vi "Emballage_BDD_GVF_DATACMD.vi"(0 "SetGet":T2=enum."get", 1 "Quantité de la commande IN":string, 5 "Cmde_Interne? IN":bool, 7 "Annuler new série (T=OK) IN":bool, 9 "No commande FAS IN":string, 11 "Error in":errorcluster caption="Error in (no error)", 12 "DATA cmde IN":T1={"n°article FAS"="12-216E-01-25 F120023 500mA 10ohm", "n° cmde FAS"="R03844/08-01.01.01", "quantité cmde"="4", "ID LIG cmde"="225540", "n° cmde client"="120565              ", "nom client"="Fluid Automat. Systems GmbH", "n° article client"="21088", "indice revision client"="      ", "société de facturation"="FAS Medic SA                            ", "langue a utiliser"="ALL"}) -> (3 "Quantité de la commande OUT":string, 4 "Quantité de la commande OUT":i32, 6 "Cmde_Interne? OUT":bool, 8 "Annuler new série (T=OK) OUT":bool, 10 "No commande FAS OUT":string, 13 "NO_ARTICLE_JDE":string, 14 "DATA cmde OUT":T1={"n°article FAS"="12-216E-01-25 F120023 500mA 10ohm", "n° cmde FAS"="R03844/08-01.01.01", "quantité cmde"="4", "ID LIG cmde"="225540", "n° cmde client"="120565              ", "nom client"="Fluid Automat. Systems GmbH", "n° article client"="21088", "indice revision client"="      ", "société de facturation"="FAS Medic SA                            ", "langue a utiliser"="ALL"}, 15 "Error out":errorcluster)   [LabVIEW 2020]
uses:
  Modules/FS/60_FS_Controles/60_FS_SetGet.ctl
panel:
  # "IN"
  # "OUT"
  # "#LTI 20180719:\ncommande interne pas utilisée"
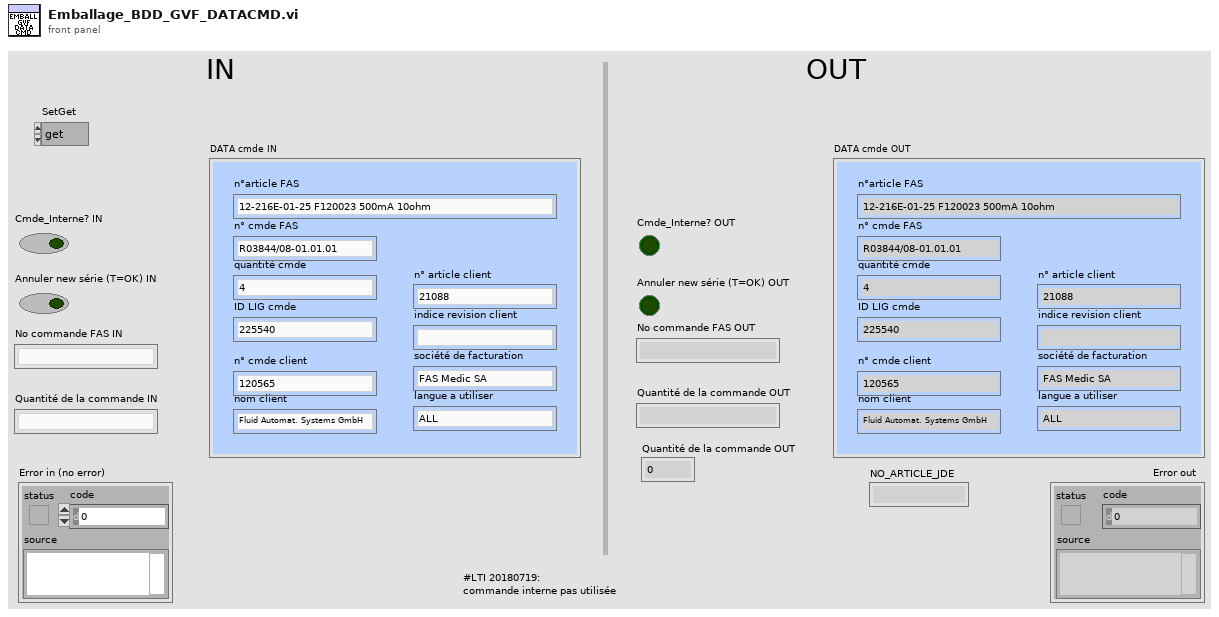
[diagram p1: front panel]
types:
  T1 = typedef "DATA commande.ctl" = cluster{"n°article FAS":string, "n° cmde FAS":string, "quantité cmde":string, "ID LIG cmde":string, "n° cmde client":string, "nom client":string, "n° article client":string, "indice revision client":string, "société de facturation":string, "langue a utiliser":string}
  T2 = typedef "60_FS_SetGet.ctl" = enum16{"set", "get"}
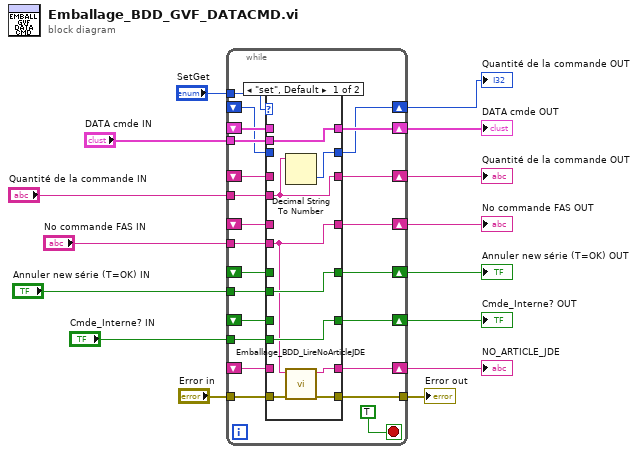
[diagram p0: block diagram]
diagram:
  n1 = while {
    tunnel: "SetGet" -> [w37]
    tunnel: "Cmde_Interne? IN" -> [w35]
    tunnel: "Annuler new série (T=OK) IN" -> [w33]
    tunnel: "No commande FAS IN" -> [w31]
    tunnel: "Quantité de la commande IN" -> [w29]
    tunnel: "DATA cmde IN" -> [w27]
    shift-right: [w36] -> w14
    shift-left: _ -> [w22]
    shift-right: [w34] -> w12
    shift-left: _ -> [w23]
    shift-right: [w32] -> w10
    shift-left: _ -> [w24]
    shift-right: [w30] -> w8
    shift-left: _ -> [w25]
    shift-right: [w28] -> w6
    shift-left: _ -> [w26]
    shift-right: [w21] -> w4
    shift-left: _ -> [w20]
    tunnel: "Error in" -> [w19]
    tunnel: [w18] -> w2
    shift-right: [w17] -> w1
    shift-left: _ -> [w16]
    stop <- TRUE stop-if-true
    n2 = case shown="\"set\", Default" w37 {
      tunnel: [w47 w51] -> w36
      tunnel: w35 -> [w47 _]
      tunnel: [w46 w52] -> w34
      tunnel: w33 -> [w46 _]
      tunnel: [w39 w53] -> w32
      tunnel: w31 -> [w39 _]
      tunnel: [w44 w54] -> w30
      tunnel: w29 -> [w44 _]
      tunnel: [w45 w55] -> w28
      tunnel: w27 -> [w45 _]
      tunnel: w26 -> [_ w55]
      tunnel: w25 -> [_ w54]
      tunnel: w24 -> [_ w53]
      tunnel: w23 -> [_ w52]
      tunnel: w22 -> [_ w51]
      tunnel: [w43 w50] -> w21
      tunnel: w20 -> [_ w50]
      tunnel: w19 -> [w42 w48]
      tunnel: [w41 w48] -> w18
      tunnel: [w40 w49] -> w17
      tunnel: w16 -> [_ w49]
      frame "set", Default {
        n3 = Decimal String To Number(string=w44) -> (number=w43:i32)  [unwired: 2 in, 1 out]
        n4 = call "Emballage_BDD_LireNoArticleJDE.vi"("error in"=w42, "NO_CDEVAL"=w39) -> ("error out"=w41:errorcluster, "NO_ARTICLE_JDE"=w40:string)  [unwired: 7 in, 1 out]
      }
      frame "get" {
      }
    }
  }
  "Error out" <- w2
  "Cmde_Interne? OUT" <- w14
  "Annuler new série (T=OK) OUT" <- w12
  "No commande FAS OUT" <- w10
  "DATA cmde OUT" <- w6
  "Quantité de la commande OUT" <- w8
  "Quantité de la commande OUT" <- w4
  "NO_ARTICLE_JDE" <- w1
